vi "UpdateDrawingSize.vi"(0 "reference in":refnum<class "LcPictureBox.lvclass">, 2 "WidthMargin(px)":i32, 3 "HeightMargin(px)":i32, 5 "Error In":errorcluster) -> (14 "reference out":refnum<class "LcPictureBox.lvclass">, 19 "Error Out":errorcluster)   [LabVIEW 2020, in "LcPictureBox.lvclass"]
doc: "You need to call this once the drawing area size haev changed (e.g. after the FP have been resixed).\nAlso you need to do a Redraw of all the drawn content"
uses:
  LcPictureBox.lvclass
  System.Drawing
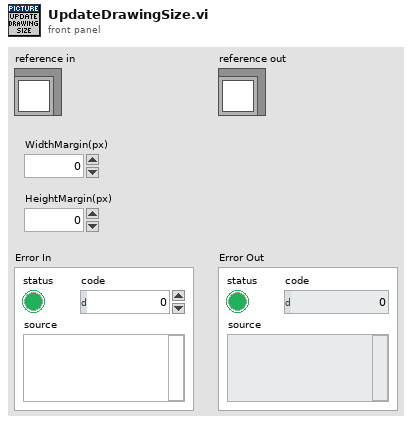
[diagram p1: front panel]
types:
  T1 = typedef "LcPictureBox.lvclass/ObjectAttributes.ctl" = cluster{"PictureBox":refnum<k24>, "ImageSize":cluster{"Width":i32, "Height":i32}, "PenMemory":map{cluster{"Alpha(100%)":dbl, "Color(Black)":u32, "Pen(Width=1, Solid)":T2}, refnum<k24>}, "GraphicsRef":refnum<k24>, "BrushMemory":map{cluster{"Alpha(100%)":dbl, "Color(Black)":u32}, refnum<k24>}, "Images":refnum<k24>[], "ImageIndex":i32, "BgColor(None)":u32, "LoadedImages":map{string, cluster{"ImageOut":refnum<k24>, "ImageSize":cluster{"Width":i32, "Height":i32}}}, "ColorsMemory":map{cluster{"Alpha(100%)":dbl, "Color(Black)":u32}, refnum<k24>}, "CacheSize":i32, "PictureBoxActiveXReference":refnum<vi>, "Scale":sgl, "Offset":cluster{"x":sgl, "y":sgl}, "zoom_center":cluster{"X":i32, "Y":i32}, "ImagesCreated":refnum<k24>[]}
  T2 = typedef "LcPictureBox.lvclass/Pen.ctl" = cluster{"Width":u16, "Style":enum32{"Solid", "Dash", "Dot", "DashDot", "DashDotDot"}}
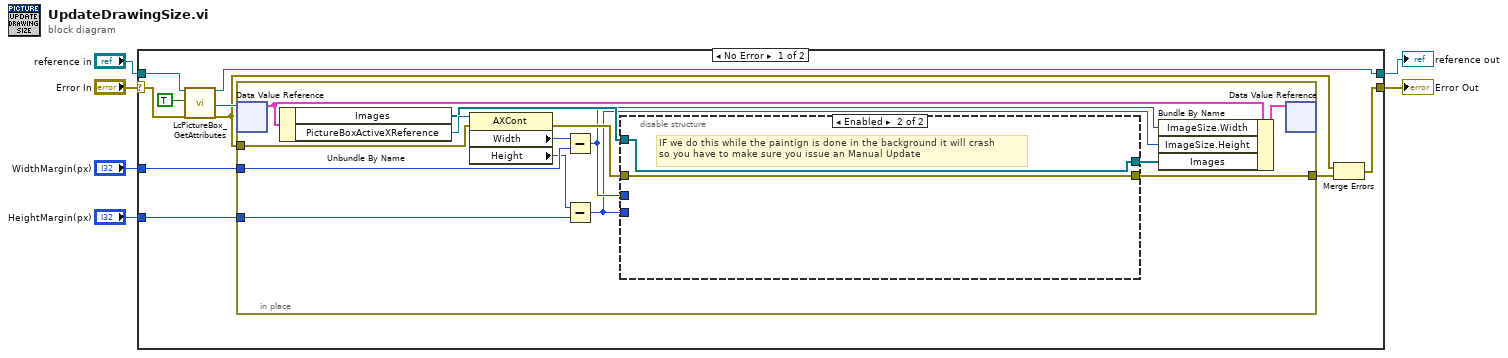
[diagram p0: block diagram]
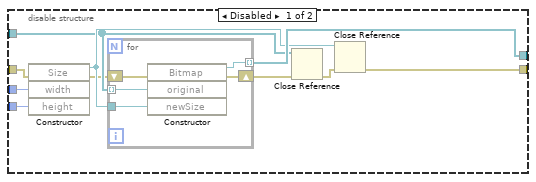
[diagram p2: hidden frame]
diagram:
  n1 = case shown="No Error" "Error In" {
    selector: "Error In" -> [w15 w49]
    tunnel: [w13 w49] -> w5
    tunnel: [w14 w48] -> w3
    tunnel: "reference in" -> [w16 w48]
    tunnel: "WidthMargin(px)" -> [w8 _]
    tunnel: "HeightMargin(px)" -> [w7 _]
    frame No Error {
      n2 = call "LcPictureBox_GetAttributes.vi"("reference in"=w16, "OnlyGetDvrReference(False)"=TRUE, "error in (no error)"=w15) -> ("reference out"=w14:refnum<class "LcPictureBox.lvclass">, "DataRef"=w12:refnum<data-value>, "error out"=w10:errorcluster)  [unwired: 13 in, 1 out]
      n3 = in-place {
        in-place-border: w10 -> [w27]
        in-place-border: [w25] -> w9
        in-place-border: w8 -> [w21]
        in-place-border: w7 -> [w19]
        n4 = in-place-dvr #1(w12) -> (w28:T1)  [unwired: 1 out]
        n5 = Unbundle By Name(w28) -> ("Images"=w24:refnum<k24>[], "PictureBoxActiveXReference"=w29:refnum<vi>)
        n6 = property on="Property Node" class="AXCont"(reference=w29, error in=w27) -> (error out=w23:errorcluster, "Width"=w22:u32, "Height"=w18:u32)  [unwired: 1 out]
        n7 = Subtract(x=w22, y=w21) -> (x-y=w20:u32)
        n8 = Subtract(x=w18, y=w19) -> (x-y=w17:u32)
        n9 = disable-structure shown="Enabled" {
          disable-tunnel: [w40 w47] -> w26
          disable-tunnel: [w38 w46] -> w25
          disable-tunnel: w24 -> [w37 w47]
          disable-tunnel: w17 -> [w34 _]
          disable-tunnel: w20 -> [w33 _]
          disable-tunnel: w23 -> [w32 w46]
          frame Disabled {
            n10 = constructor class="Size"(error in=w32, "width"=w33, "height"=w34) -> (reference out=w39:refnum<k24>, error out=w31:errorcluster)  [unwired: 2 in, 3 out]
            n11 = for {
              tunnel: w39 -> [w41]
              tunnel: w37 -> [w44] mode=indexing
              tunnel: [w43] -> w40 mode=indexing
              shift-right: [w42] -> w36
              shift-left: w31 -> [w45]
              n12 = constructor class="Bitmap"(error in=w45, "original"=w44, "newSize"=w41) -> (reference out=w43:refnum<k24>, error out=w42:errorcluster)  [unwired: 2 in, 3 out]
            }
            n13 = Close Reference(reference=w37, error in (no error)=w36) -> (error out=w35:errorcluster)
            n14 = Close Reference(reference=w39, error in (no error)=w35) -> (error out=w38:errorcluster)
          }
          frame Enabled {
            # "IF we do this while the paintign is done in the background it will crash\nso you have to make sure you issue an Manual Update"
          }
        }
        n15 = Bundle By Name(cluster=w28, "ImageSize.Width"=w20, "ImageSize.Height"=w17, "Images"=w26) -> (w30:T1)
        n16 = in-place-dvr #1(w30) -> ()  [unwired: 2 out]
      }
      n17 = Merge Errors(w10, w9) -> (w13:errorcluster)
    }
    frame Error {
    }
  }
  "Error Out" <- w5
  "reference out" <- w3
